vi "bool to msgpack.vi"(11 "Boolean":bool=TRUE) -> (3 "msgpack":u8[](array[numeric]) format="%x")   [LabVIEW 2020, in "wamplv.lvlib" / "MessagePack.lvclass"]
uses:
  MessagePack.lvclass
  Format bytes.ctl
  MessagePack.lvclass/MessagePack.ctl
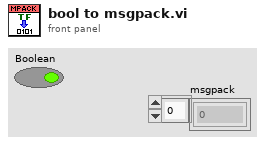
[diagram p1: front panel]
types:
  T1 = typedef "wamplv.lvlib/MessagePack.lvclass/Format bytes.ctl" = u8
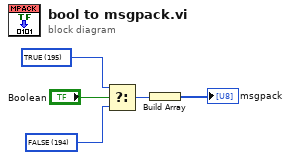
[diagram p0: block diagram]
diagram:
  w1 = T1 194 items=["nil"=192, "UINT8"=204, "UINT16"=205, "UINT32"=206, "UINT64"=207, "INT8"=208, "INT16"=209, "INT32"=210, "INT64"=211, "FALSE"=194, "TRUE"=195, "SGL"=202, "DBL"=203] ("Format byte")
  w2 = T1 195 items=["nil"=192, "UINT8"=204, "UINT16"=205, "UINT32"=206, "UINT64"=207, "INT8"=208, "INT16"=209, "INT32"=210, "INT64"=211, "FALSE"=194, "TRUE"=195, "SGL"=202, "DBL"=203] ("Format byte")
  n1 = Select(t=w2, s="Boolean", f=w1) -> (s? t:f=w3:T1)
  n2 = Build Array(w3) -> (→"msgpack":T1[])
